vi "JL - Verify Blink.vi"(0 "GEA2 Reference In":refnum<k24>, 1 "SSD":string, 2 "Blinking LED":T1, 5 "Initial Timeout (s)":dbl, 7 "Retry Count":i32, 9 "Max Blink Rate (sec)":dbl, 11 "Error In":errorcluster) -> (4 "GEA2 Reference Out":refnum<k24>, 6 "Pass/Fail?":bool, 8 "Report Text":string, 10 "Blink Times (s)":dbl[](array[numeric]), 15 "Error Out":errorcluster)   [LabVIEW 2016]
doc: "This VI is used to verify that a particular LED is blinking on the HEUI."
uses:
  Q:/Common/DLLs/GEA3/GeaCommunication.dll
  Common/DLLs/GEA3/GeaCommunication.dll
  type defs/JL_Display_Blink.ctl
  Common/LabVIEW GEA2 Toolkit/LabVIEW_GEA2_Toolkit.lvlibp/type defs/Source_Destination.ctl
  Common/LabVIEW GEA2 Toolkit/LabVIEW_GEA2_Toolkit.lvlibp
panel:
  in  "Standalone":bool
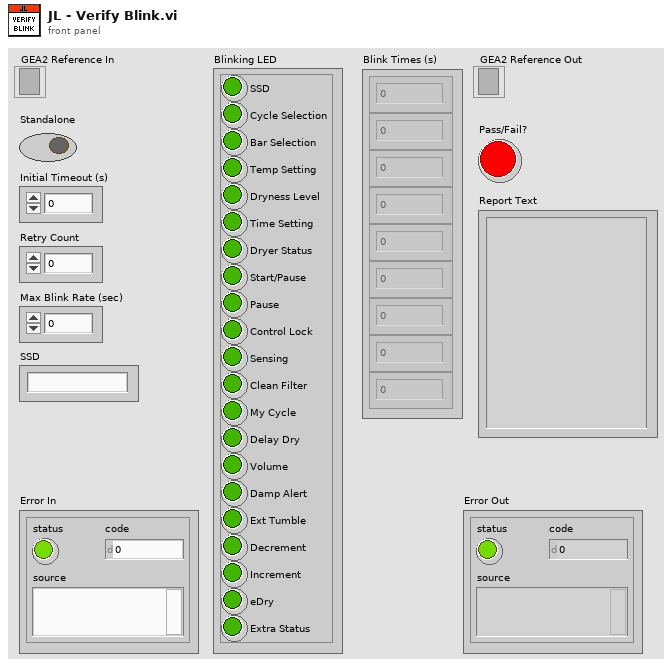
[diagram p1: front panel]
types:
  T1 = typedef "JL_Display_Blink.ctl" = cluster{"SSD":bool, "Cycle Selection":bool, "Bar Selection":bool, "Temp Setting":bool, "Dryness Level":bool, "Time Setting":bool, "Dryer Status":bool, "Start/Pause":bool, "Pause":bool, "Control Lock":bool, "Sensing":bool, "Clean Filter":bool, "My Cycle":bool, "Delay Dry":bool, "Volume":bool, "Damp Alert":bool, "Ext Tumble":bool, "Decrement":bool, "Increment":bool, "eDry":bool, "Extra Status":bool}
  T2 = typedef "LabVIEW_GEA2_Toolkit.lvlibp/Source_Destination.ctl" = cluster{"Source":u8, "Destination":u8}
  T3 = typedef "JL Display Care.ctl" = cluster{"SSD":bool, "Cycle Selection":bool, "Bar Selection":bool, "Temp Setting":bool, "Dryness Level":bool, "Time Setting":bool, "Dryer Status":bool, "Start/Pause":bool, "Pause":bool, "Control Lock":bool, "Sensing":bool, "Clean Filter":bool, "My Cycle":bool, "Delay Dry":bool, "Volume":bool, "Damp Alert":bool, "Ext Tumble":bool, "Decrement":bool, "Increment":bool, "eDry":bool, "Extra Status":bool}
  T4 = typedef "JL Display.ctl" = cluster{"SSD":string, "Cycle Selection":T5, "Bar Selection":T6, "Temp Setting":T7, "Dryness Level":T8, "Time Setting":T9, "Dryer Status":T10, "Start/Pause":bool, "Pause":bool, "Control Lock":bool, "Sensing":bool, "Clean Filter":bool, "My Cycle":bool, "Delay Dry":bool, "Volume":bool, "Damp Alert":bool, "Ext Tumble":bool, "Decrement":bool, "Increment":bool, "eDry":bool, "Extra Status":bool}
  T5 = typedef "Cycle Selection Enum.ctl" = enum16{"Cycle 0", "Cycle 1", "Cycle 2", "Cycle 3", "Cycle 4", "Cycle 5", "Cycle 6", "Cycle 7", "Cycle 8", "Cycle 9", "Cycle 10", "Cycle 11", "Cycle 12", "Cycle 13", "Off", "*Invalid"}
  T6 = typedef "Bar Enum.ctl" = enum16{"Bar 1", "Bar 2", "Bar 3", "Bar 4", "Bar 5", "Off", "*Incorrect*"}
  T7 = typedef "Temp Setting Enum.ctl" = enum16{"Off", "No Heat", "Extra Low", "Low", "Medium", "High", "*Incorrect*"}
  T8 = typedef "Dryness Enum.ctl" = enum16{"Off", "Damp", "Less Dry", "Dry", "More Dry", "Extra Dry", "*Incorrect*"}
  T9 = typedef "Time Enum.ctl" = enum16{"Off", "Default Time 1", "Default Time 2", "Default Time 3", "Default Time 4", "Default Time 5", "*Incorrect*"}
  T10 = typedef "Status Enum.ctl" = enum16{"Status 1", "Status 2", "Status 3", "Status 4", "Status 5", "Status 6", "Off", "*Incorrect*"}
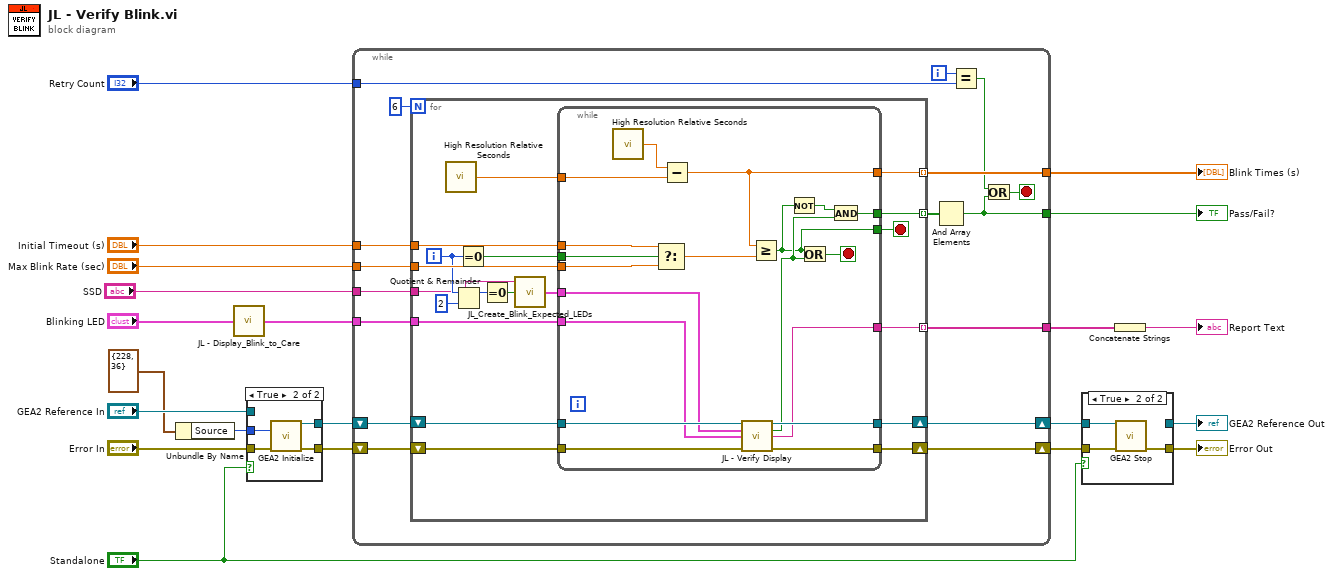
[diagram p0: block diagram]
diagram:
  n1 = Unbundle By Name(T2 {"Source"=228, "Destination"=36} ("GEA Inputs")) -> ("Source"=w20:u8)
  n2 = call "JL - Display_Blink_to_Care.vi"("JL_Display_Blink"="Blinking LED") -> ("Care?"=w3:T3)  [unwired: 14 in]
  n3 = case shown="True" "Standalone" {
    tunnel: "Error In" -> [w23 w27]
    tunnel: w20 -> [_ w26]
    tunnel: [w22 w25] -> w12
    tunnel: [w23 w24] -> w11
    tunnel: "GEA2 Reference In" -> [w22 _]
    frame False {
    }
    frame True {
      n4 = call "GEA2 Initialize.vi"("Source Address"=w26, "error in"=w27) -> ("GEA2 Reference Out"=w25:refnum<k24>, "error out"=w24:errorcluster)  [unwired: 11 in, 1 out]
    }
  }
  n5 = while {
    tunnel: "Max Blink Rate (sec)" -> [w44]
    tunnel: [w33] -> w6
    tunnel: [w43] -> w13
    tunnel: w3 -> [w38]
    tunnel: "Initial Timeout (s)" -> [w37]
    shift-right: [w40] -> w10
    shift-left: w12 -> [w42]
    shift-right: [w39] -> w9
    shift-left: w11 -> [w41]
    tunnel: [w36] -> w7
    tunnel: "Retry Count" -> [w30]
    tunnel: "SSD" -> [w28]
    i -> [w31]
    stop <- w32 stop-if-true
    n6 = for {
      N: 6 -> [_]
      shift-right: [w62] -> w39
      shift-left: w41 -> [w63]
      shift-right: [w61] -> w40
      shift-left: w42 -> [w60]
      tunnel: w44 -> [w58]
      tunnel: [w56] -> w35 mode=indexing
      tunnel: [w53] -> w36 mode=indexing
      tunnel: [w57] -> w43 mode=indexing
      tunnel: w38 -> [w52]
      tunnel: w37 -> [w54]
      tunnel: w28 -> [w45]
      i -> [w46]
      stop <- w47 stop-if-true
      n7 = call <vilib>:"High Resolution Relative Seconds.vi"() -> ("relative seconds"=w59:dbl)
      n8 = Quotient & Remainder(x=w46, y=2) -> (x-y*floor(x/y)=w50:i32)  [unwired: 1 out]
      n9 = Equal To 0?(x=w46) -> (x = 0?=w55:bool)
      n10 = Equal To 0?(x=w50) -> (x = 0?=w49:bool)
      n11 = call "JL_Create_Blink_Expected_LEDs.vi"("SSD"=w45, "Boolean"=w49) -> ("Expected LEDs Out"=w48:T4)  [unwired: 13 in]
      n12 = while {
        tunnel: w63 -> [w70]
        tunnel: [w69] -> w62
        tunnel: [w71] -> w61
        tunnel: w60 -> [w72]
        tunnel: w59 -> [w81]
        tunnel: w58 -> [w76]
        tunnel: [w79] -> w56
        tunnel: [w80] -> w57
        tunnel: w55 -> [w73]
        tunnel: w52 -> [w68]
        tunnel: w54 -> [w77]
        tunnel: [w67] -> w53
        tunnel: w48 -> [w64]
        tunnel: [w65] -> w47
        stop <- w78 stop-if-true
        n13 = call <vilib>:"High Resolution Relative Seconds.vi"() -> ("relative seconds"=w82:dbl)
        n14 = Select(t=w77, s=w73, f=w76) -> (s? t:f=w75:dbl)
        n15 = Subtract(x=w82, y=w81) -> (x-y=w80:dbl)
        n16 = call "JL - Verify Display.vi"("GEA2 Reference In"=w72, "Expected LEDs"=w64, "Care?"=w68, "Error In"=w70) -> ("GEA2 Reference Out"=w71:refnum<k24>, "Pass/Fail?"=w66:bool, "Report Text"=w67:string, "Error Out"=w69:errorcluster)  [unwired: 8 in]
        n17 = Greater Or Equal?(x=w80, y=w75) -> (x >= y?=w65:bool)
        n18 = Not(x=w65) -> (.not. x?=w74:bool)
        n19 = Or(x=w65, y=w66) -> (x .or. y?=w78:bool)
        n20 = And(x=w74, y=w66) -> (x .and. y?=w79:bool)
      }
    }
    n21 = And Array Elements(Boolean array=w35) -> (logical AND=w33:bool)
    n22 = Equal?(x=w31, y=w30) -> (x = y?=w34:bool)
    n23 = Or(x=w34, y=w33) -> (x .or. y?=w32:bool)
  }
  "Pass/Fail?" <- w6
  "Blink Times (s)" <- w13
  n24 = case shown="True" "Standalone" {
    tunnel: w9 -> [w84 w87]
    tunnel: [w84 w86] -> w18
    tunnel: w10 -> [w83 w85]
    tunnel: [w83 _] -> w16
    frame False {
    }
    frame True {
      n25 = call "GEA2 Stop.vi"("GEA2 Reference In"=w85, "Error In"=w87) -> ("Error Out"=w86:errorcluster)  [unwired: 13 in]
    }
  }
  "GEA2 Reference Out" <- w16
  "Error Out" <- w18
  n26 = Concatenate Strings(w7) -> (→"Report Text":string)
